vi "Test USB4671.vi"() -> ()   [LabVIEW 2017]
panel:
  in  "stop":bool
  out "DO error out":errorcluster
  out "DI error out":errorcluster
  in  "DO":bool[][](array[boolean])
  out "DI":bool[][](array[boolean])
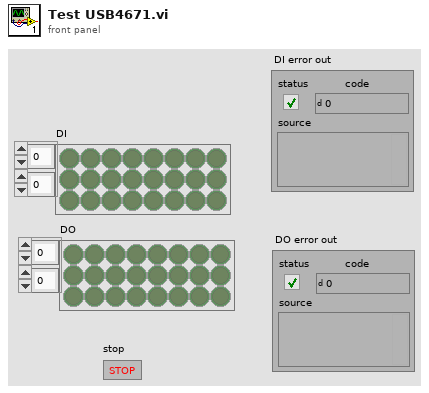
[diagram p1: front panel]
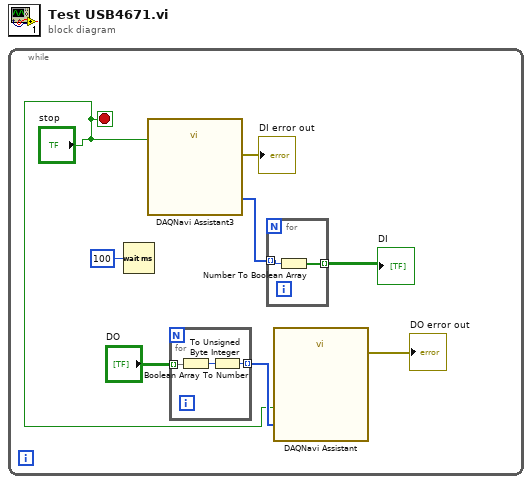
[diagram p0: block diagram]
diagram:
  n1 = while {
    stop <- "stop" stop-if-true
    n2 = Wait (ms)(milliseconds to wait=u32 100) -> ()  [unwired: 1 out]
    n3 = call "DAQNavi Assistant3"("stop(true)"="stop") -> ("error out"=→"DI error out":errorcluster, "dataOut(U8Array)"=w4:u8[])  [unwired: 25 in]
    n4 = for {
      tunnel: [w10] -> w3 mode=indexing
      tunnel: "DO" -> [w9] mode=indexing
      n5 = Boolean Array To Number(Boolean array=w9) -> (number=w11:u32)
      n6 = To Unsigned Byte Integer(number=w11) -> (unsigned 8bit integer=w10:u8)
    }
    n7 = for {
      tunnel: [w13] -> w8 mode=indexing
      tunnel: w4 -> [w12] mode=indexing
      n8 = Number To Boolean Array(number=w12) -> (Boolean array=w13:bool[])
    }
    "DI" <- w8
    n9 = call "DAQNavi Assistant"("stop(true)"="stop", "dataIn(U8Array)"=w3) -> ("error out"=→"DO error out":errorcluster)  [unwired: 25 in]
  }
